vi "Copy_Files.vi"(8 "error in (no error)":errorcluster, 11 "Build in":refnum<class "AB_Application.lvclass">) -> (0 "error out":errorcluster, 3 "Build out":refnum<class "AB_Application.lvclass">)   [LabVIEW 2020, in "AB_Application.lvclass"]
uses:
  <vilib>/AppBuilder/AB_Classes/Application/AB_Application.lvclass
  <vilib>/AppBuilder/AB_Classes/TargetFile/AB_Targetfile.lvclass
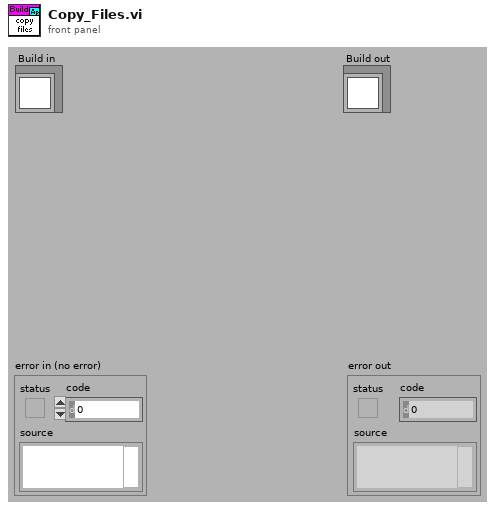
[diagram p1: front panel]
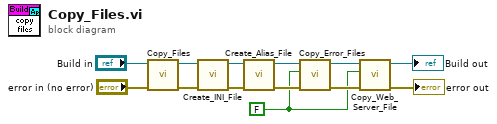
[diagram p0: block diagram]
diagram:
  w1 = FALSE ("preview only?")
  n1 = call-parent "Copy_Files.vi"("error in (no error)"="error in (no error)", "Build in"="Build in") -> ("error out"=w10:errorcluster, "Build out"=w11:refnum<class "AB_Application.lvclass">)  [unwired: 8 out]
  n2 = call-dynamic "Create_INI_File.vi"("error in (no error)"=w10, "AB_Application in"=w11) -> ("error out"=w8:errorcluster, "AB_Application out"=w9:refnum<class "AB_Application.lvclass">)  [unwired: 8 out]
  n3 = call-dynamic "Create_Alias_File.vi"("error in (no error)"=w8, "AB_Application in"=w9) -> ("error out"=w7:errorcluster, "AB_Application out"=w6:refnum<class "AB_Application.lvclass">)  [unwired: 8 out]
  n4 = call-dynamic "Copy_Error_Files.vi"("error in (no error)"=w7, "preview only?"=w1, "AB_Application in"=w6) -> ("error out"=w3:errorcluster, "AB_Application out"=w5:refnum<class "AB_Application.lvclass">)  [unwired: 7 out]
  n5 = call-dynamic "Copy_Web_Server_File.vi"("error in (no error)"=w3, "preview only?"=w1, "AB_Application in"=w5) -> ("error out"=→"error out":errorcluster, "AB_Application out"=→"Build out":refnum<class "AB_Application.lvclass">)  [unwired: 7 out]
